vi "UIRef.vi"(8 "error in":errorcluster, 11 "fixed channel editor in":refnum<class "AppStateMachine editor node.lvclass">) -> (0 "error out":errorcluster, 2 "VI refnum":refnum<vi>, 3 "fixed channel editor out":refnum<class "AppStateMachine editor node.lvclass">)   [LabVIEW 2017, in "AppStateMachine editor node.lvclass"]
uses:
  AppStateMachine editor node.lvclass
  configUI.vi
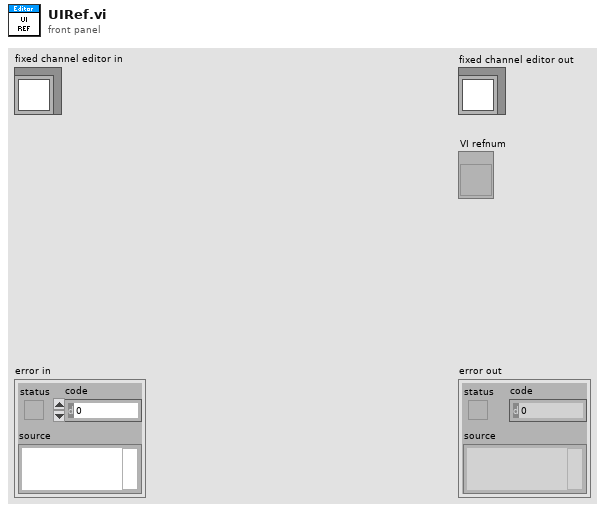
[diagram p1: front panel]
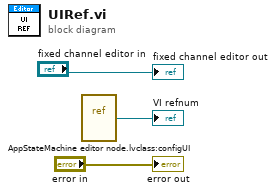
[diagram p0: block diagram]
diagram:
  n1 = vi-ref "AppStateMachine editor node.lvclass:configUI.vi"() -> (→"VI refnum":refnum<vi>)
  "error out" <- "error in"
  "fixed channel editor out" <- "fixed channel editor in"
